vi "TestSortedRecipeFOlderData.vi"() -> ()   [LabVIEW 2022 SP3]
uses:
  Controls/RecipesFolderSummary--Cluster.ctl
  Controls/DLP RecipeTypesData--Cluster.ctl
  Controls/RecipeInfo--Cluster.ctl
panel:
  out "Type":string
  in  "error in (no error)":errorcluster
  in  "OK":bool
  out "found":bool
  in  "RecipeFolderPath":path
  in  "Recipe":u16(ring) items=["25x29 Token Recipe DOE001"]
  in  "Product":u16(ring) items=["25x29 Token", "C30v3.2"]
  in  "RecipeType":u16(ring) items=["PrintDesign", "Calibration"]
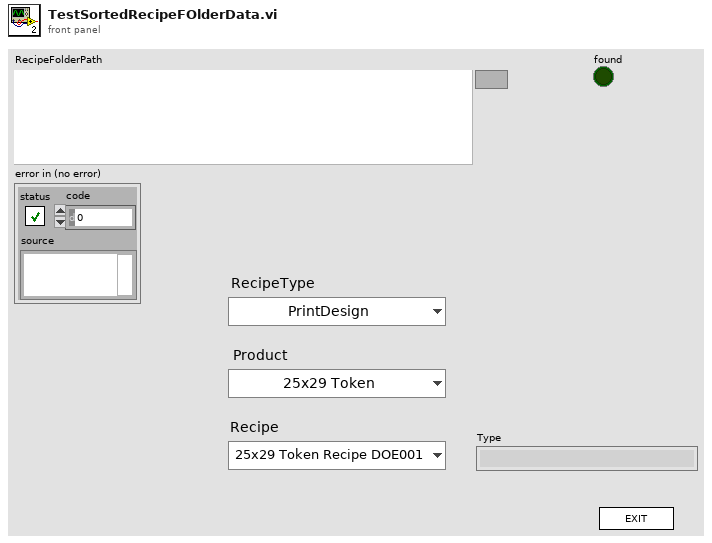
[diagram p1: front panel]
types:
  T1 = typedef "RecipesFolderSummary--Cluster.ctl" = cluster{"Products":string[], "RecipeTypes":string[]}
  T2 = typedef "TD Dynamic CVT DVR--ref.ctl" = refnum<data-value>
  T3 = enum32{"Invalid", "Standard", "Closed", "Hidden", "Minimized", "Maximized"}
  T4 = enum32{"invalid app kind", "Development System", "Run Time System", "Student Edition", "Embedded LabVIEW", "Evaluation", "Custom"}
  T5 = cluster{"Core":cluster{"Current VI Reference":refnum<vi>, "Close Panel on Exit?":bool}, "Your Boolean data":bool, "dCVT DVR out":T2}
  T6 = cluster{"Current VI Reference":refnum<vi>, "Close Panel on Exit?":bool}
  T7 = typedef "DLP RecipeTypesData--Cluster.ctl" = cluster{"Product":string, "RecipePathsByProduct":path[], "RecipeNamesByProduct":string[]}
  T8 = typedef "RecipeInfo--Cluster.ctl" = cluster{"Path":path, "Type":string}
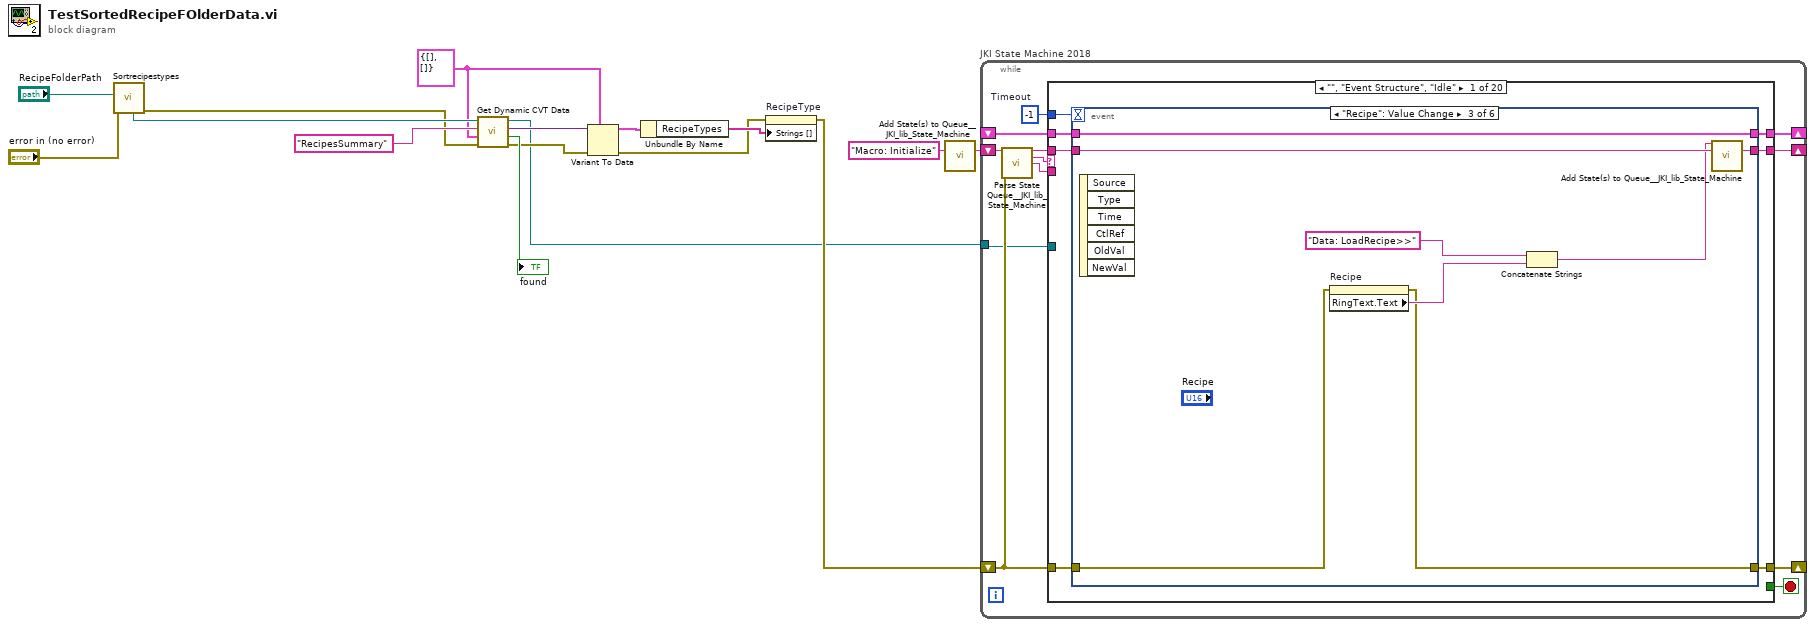
[diagram p0: block diagram]
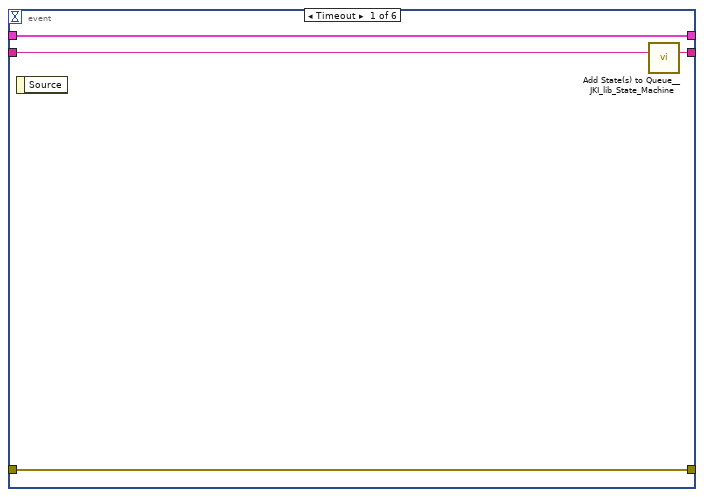
[diagram p2: hidden frame]
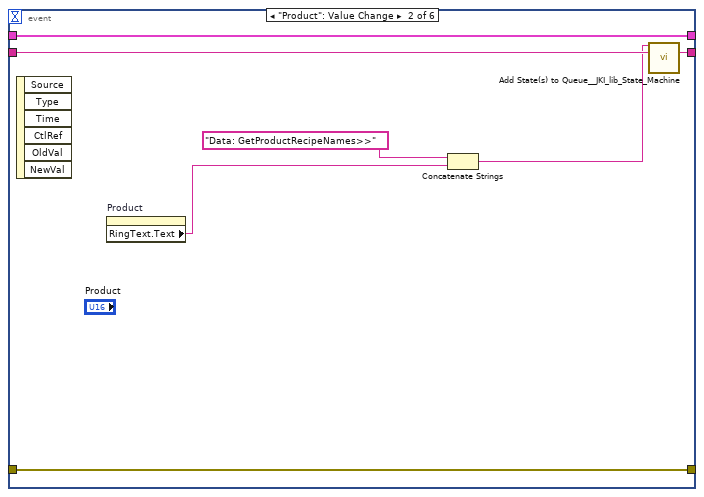
[diagram p3: hidden frame]
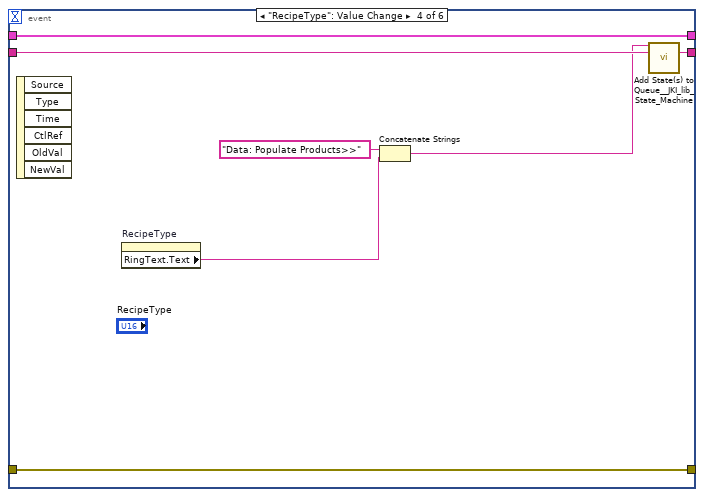
[diagram p4: hidden frame]
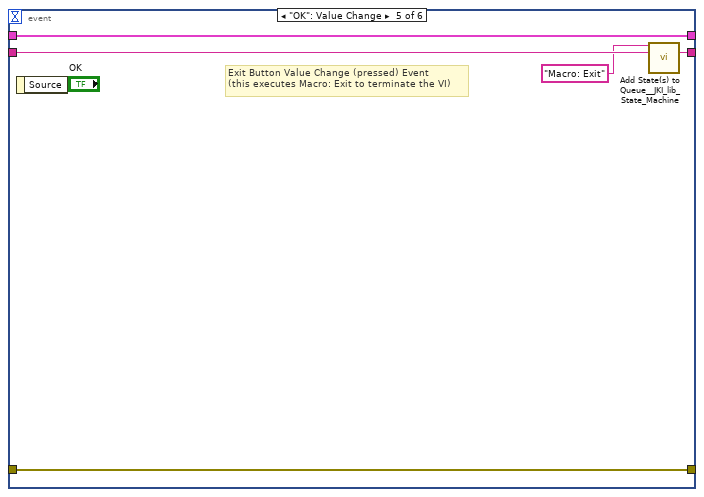
[diagram p5: hidden frame]
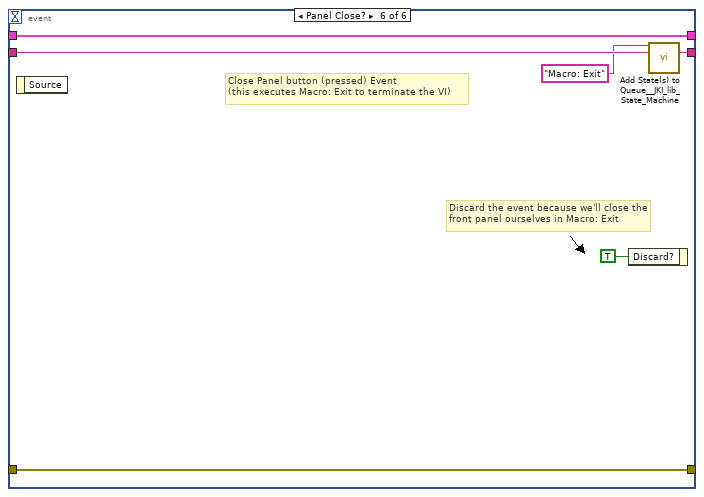
[diagram p6: hidden frame]
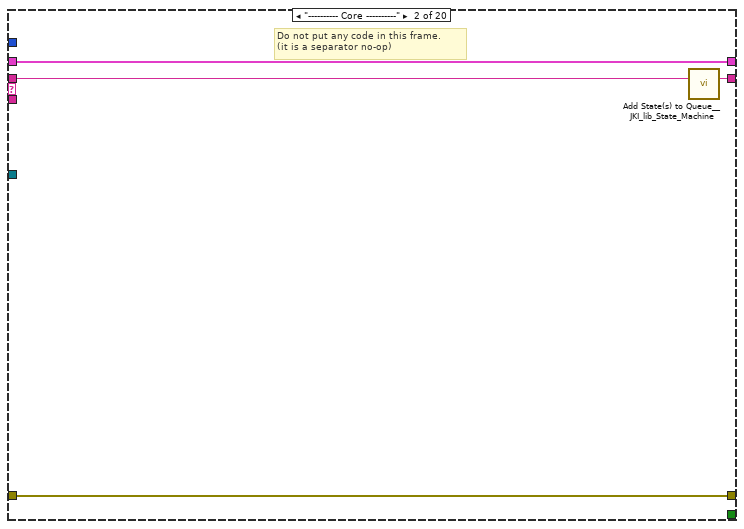
[diagram p7: hidden frame]
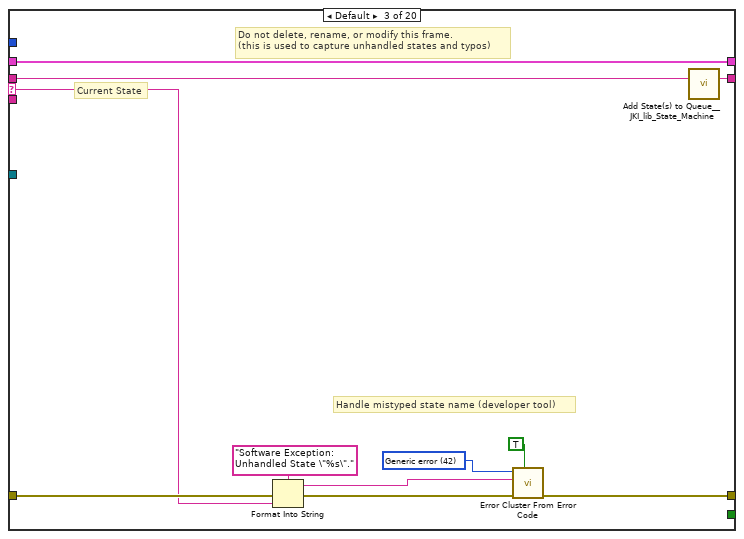
[diagram p8: hidden frame]
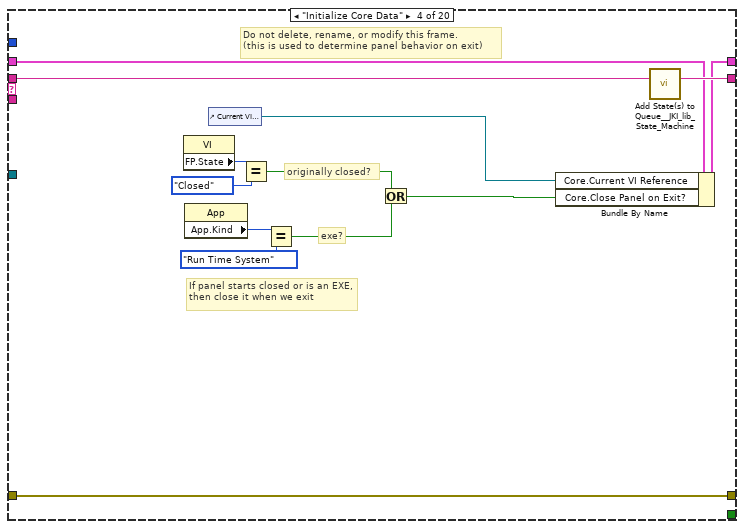
[diagram p9: hidden frame]
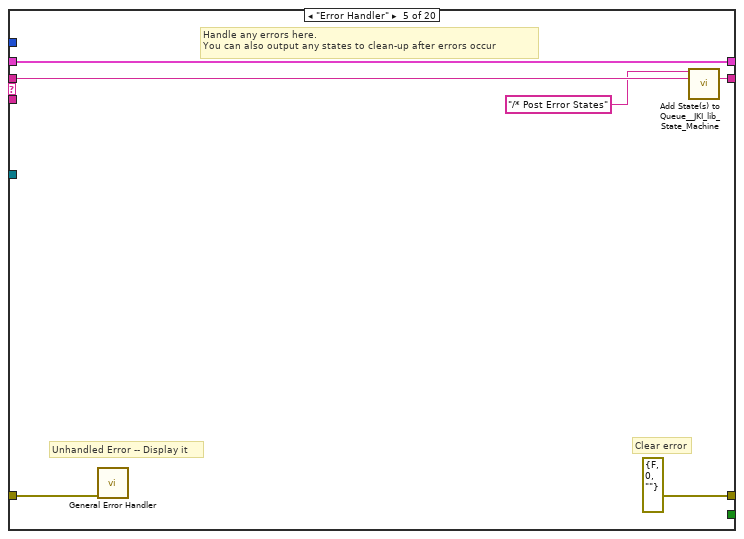
[diagram p10: hidden frame]
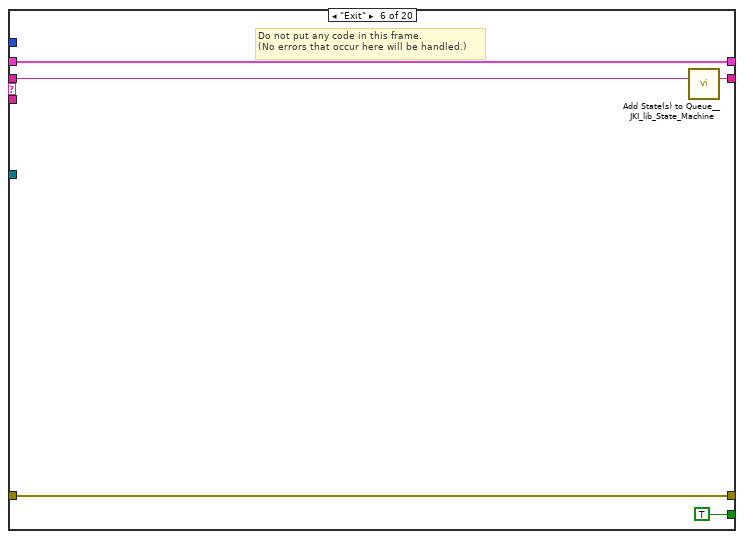
[diagram p11: hidden frame]
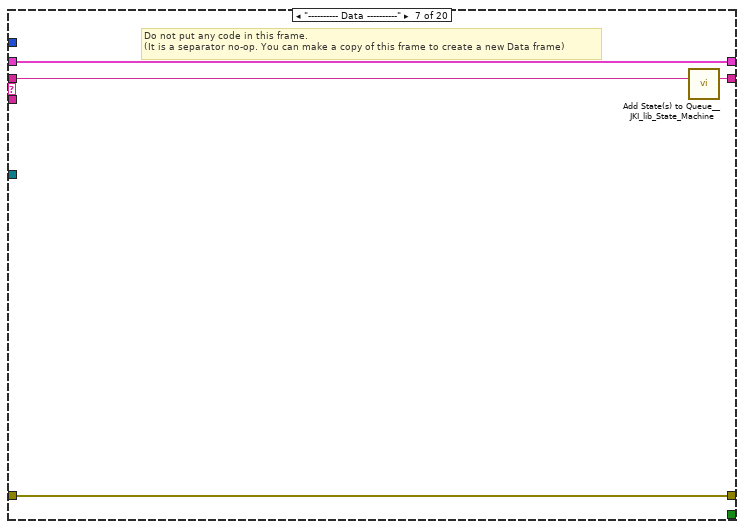
[diagram p12: hidden frame]
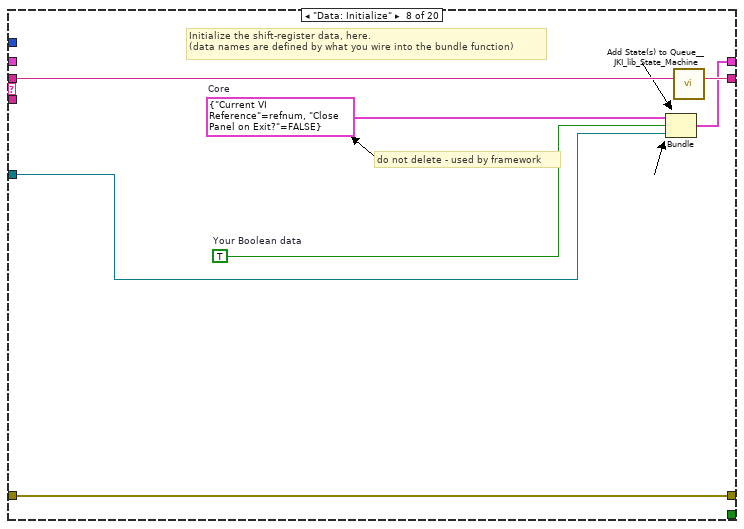
[diagram p13: hidden frame]
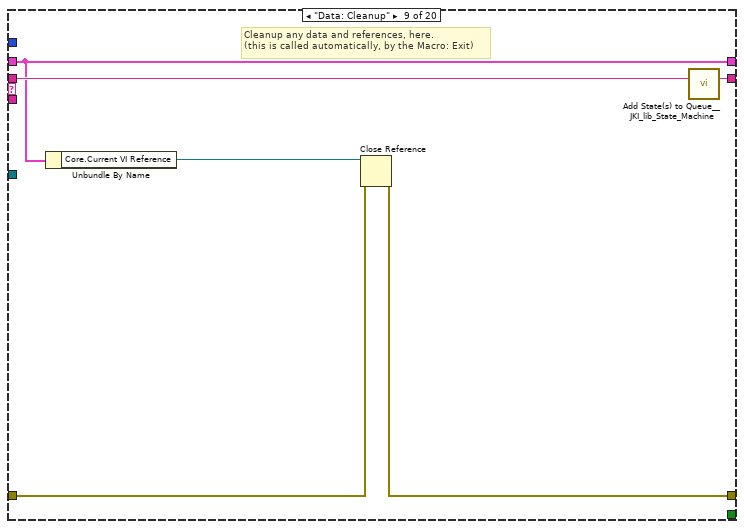
[diagram p14: hidden frame]
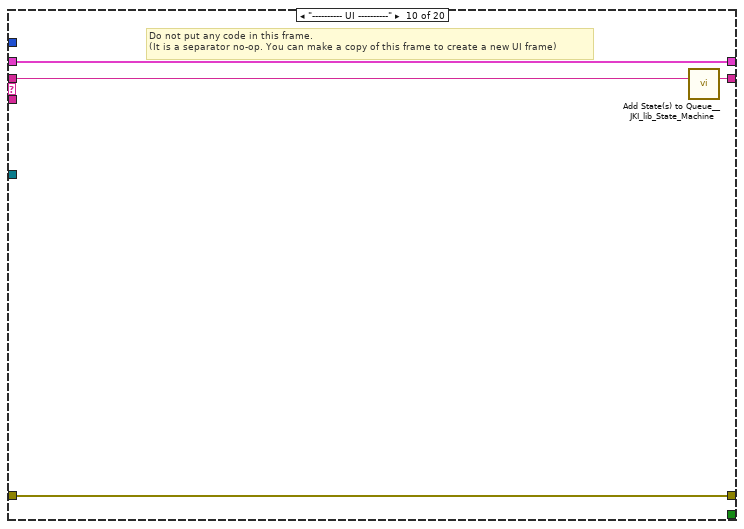
[diagram p15: hidden frame]
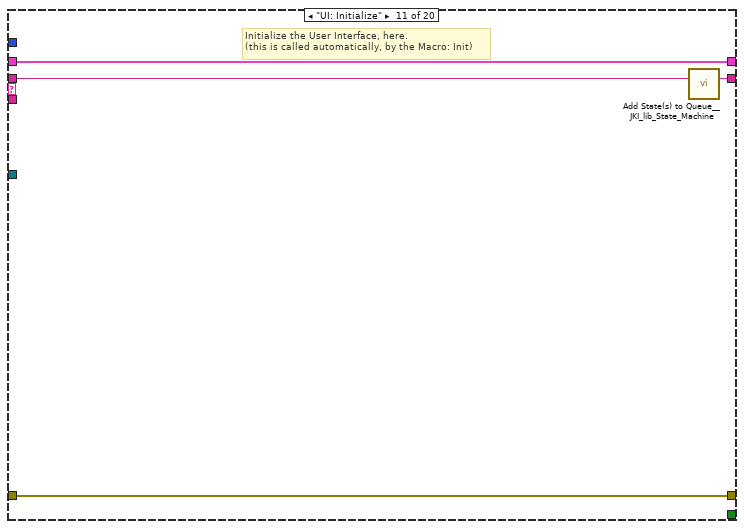
[diagram p16: hidden frame]
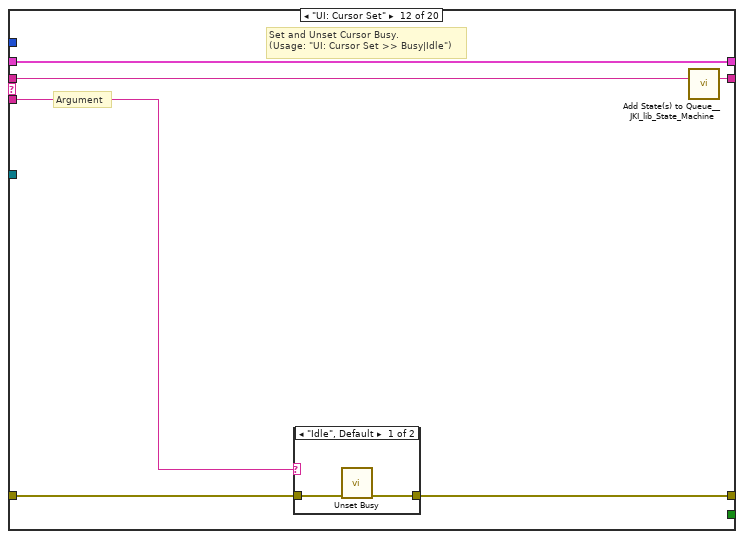
[diagram p17: hidden frame]
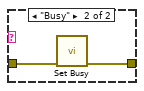
[diagram p18: hidden frame]
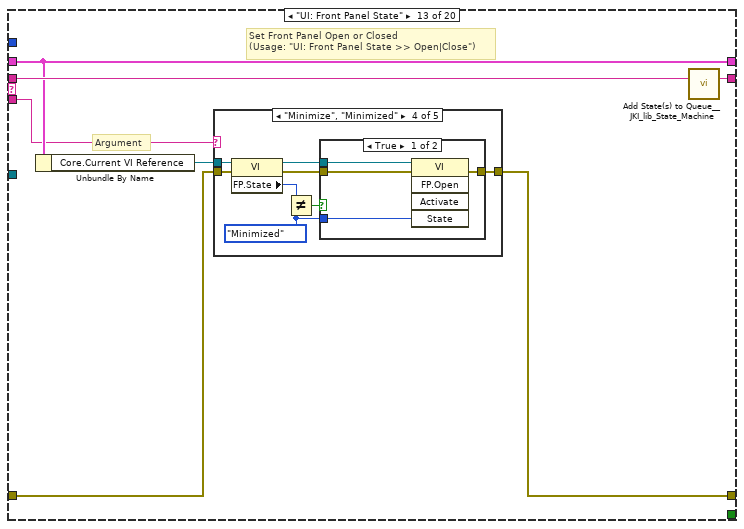
[diagram p19: hidden frame]
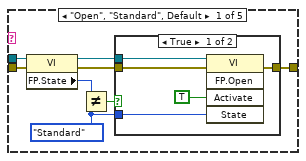
[diagram p20: hidden frame]
diagram:
  w11 = T1 {"Products"=[], "RecipeTypes"=[]}
  n1 = call "Sortrecipestypes.vi"("error in (no error)"="error in (no error)", "RecipeFolderPath"="RecipeFolderPath") -> ("error out"=w2:errorcluster, "DebugDict"=w14:T2)  [unwired: 5 in, 3 out]
  n2 = call <vilib>:"Get Dynamic CVT Data.vi"("error in (no error)"=w2, "default value (empty variant)"=w11, "DataName"="RecipesSummary", "dCVT DVR"=w14) -> ("error out"=w10:errorcluster, "found"=→"found":bool, "value"=w12:variant, "dCVT DVR out"=w4:T2)  [unwired: 4 in]
  n3 = Variant To Data(error in=w10, type=w11, Variant=w12) -> (data=w9:T1, error out=w3:errorcluster)
  n4 = Unbundle By Name(w9) -> ("RecipeTypes"=w8:string[])
  n5 = property on="RecipeType" class="Ring (strict)"(error in=w3, "Strings []"=w8) -> (error out=w5:errorcluster)  [unwired: 1 in, 1 out]
  n6 = call <vilib>:"Add State(s) to Queue__JKI_lib_State_Machine.vi"("State(s) in (\"\")"="Macro: Initialize") -> ("States Out"=w7:string)  [unwired: 14 in]
  n7 = while "JKI State Machine 2018" {
    shift-right: [w21] -> _
    shift-left: _ -> [w20]
    shift-right: [w24] -> _
    shift-left: w5 -> [w18]
    shift-right: [w23] -> _
    shift-left: w7 -> [w25]
    tunnel: w4 -> [w17]
    stop <- w22 stop-if-true
    w19 = -1  # Timeout
    n8 = call <vilib>:"Parse State Queue__JKI_lib_State_Machine.vi"("State Queue"=w25, "Error In (no error)"=w18) -> ("Remaining States"=w27:string, "Current State"=w28:string, "Arguments"=w26:string)  [unwired: 11 in]
    n9 = case shown="\"\", \"Event Structure\", \"Idle\"" w28 {
      selector: w28 -> [_ _ w77 _ _ _ _ _ _ _ _ _ _ _ _ _ _ _ _ _]
      tunnel: w27 -> [w35 w76 w81 w100 w106 w111 w115 w122 w128 w132 w136 w142 w153 w222 w227 w237 w241 w254 w268 w282]
      tunnel: w26 -> [_ _ _ _ _ _ _ _ _ _ _ w137 w147 _ _ _ _ w248 w263 w276]
      tunnel: w20 -> [w33 w73 w79 w93 w103 w109 w112 _ w123 w129 w134 w140 w149 w219 w224 w234 w238 w249 w266 w277]
      tunnel: [w32 w74 w83 w97 errorcluster {"status"=FALSE, "code"=0, "source"=""} ("error out") w108 w113 w119 w124 w130 w133 w138 w150 w220 w225 w235 w239 w243 w255 w269] -> w24
      tunnel: w18 -> [w31 w74 w82 w97 w102 w108 w113 w119 w125 w130 w133 w139 w151 w220 w225 w235 w239 w242 w261 w272]
      tunnel: [w34 w75 w80 w99 w105 w110 w114 w121 w127 w131 w135 w141 w152 w221 w226 w236 w240 w253 w267 w281] -> w23
      tunnel: [_ _ _ _ _ TRUE _ _ _ _ _ _ _ _ _ _ _ _ _ _] -> w22
      tunnel: [w30 w73 w79 w98 w103 w109 w112 w120 w123 w129 w134 w140 w149 w219 w224 w234 w238 w249 w266 w277] -> w21
      tunnel: w19 -> [w29 _ _ _ _ _ _ _ _ _ _ _ _ _ _ _ _ _ _ _]
      tunnel: w17 -> [_ _ _ _ _ _ _ w116 _ _ _ _ _ _ _ _ _ _ _ _]
      frame "", "Event Structure", "Idle" {
        n10 = event shown="[2] \"Recipe\": Value Change" {
          selector: _ -> [_ _ _ _ _ _]
          dyn-events: _ -> [_ _ _ _ _ _]
          timeout: w29 -> [_ _ _ _ _ _]
          tunnel: w35 -> [w39 w46 w54 w61 w66 w72]
          tunnel: [w38 w45 w53 w60 w65 w71] -> w34
          tunnel: w33 -> [w36 w43 w52 w58 w63 w69]
          tunnel: [w37 w44 w48 w59 w64 w70] -> w32
          tunnel: w31 -> [w37 w44 w47 w59 w64 w70]
          tunnel: [w36 w43 w52 w58 w63 w69] -> w30
          event Timeout {
            n11 = event-data() -> ()  [unwired: 1 in, 1 out]
            n12 = call <vilib>:"Add State(s) to Queue__JKI_lib_State_Machine.vi"("State(s) in (\"\")"=w39) -> ("States Out"=w38:string)  [unwired: 14 in]
          }
          event "Product": Value Change {
            n13 = event-data() -> ()  [unwired: 1 in, 6 out]
            n14 = property on="Product" class="Ring (strict)"() -> ("RingText.Text"=w42:string)  [unwired: 2 in, 2 out]
            n15 = Concatenate Strings("Data: GetProductRecipeNames>>" ("string"), w42) -> (w40:string)
            n16 = call <vilib>:"Add State(s) to Queue__JKI_lib_State_Machine.vi"("State(s) in Front (\"\")"=w40, "State(s) in (\"\")"=w46) -> ("States Out"=w45:string)  [unwired: 13 in]
          }
          event "Recipe": Value Change {
            n17 = event-data() -> ()  [unwired: 1 in, 6 out]
            n18 = property on="Recipe" class="Ring (strict)"(error in=w47) -> (error out=w48:errorcluster, "RingText.Text"=w51:string)  [unwired: 1 in, 1 out]
            n19 = Concatenate Strings("Data: LoadRecipe>>" ("string"), w51) -> (w49:string)
            n20 = call <vilib>:"Add State(s) to Queue__JKI_lib_State_Machine.vi"("State(s) in Front (\"\")"=w49, "State(s) in (\"\")"=w54) -> ("States Out"=w53:string)  [unwired: 13 in]
          }
          event "RecipeType": Value Change {
            n21 = event-data() -> ()  [unwired: 1 in, 6 out]
            n22 = property on="RecipeType" class="Ring (strict)"() -> ("RingText.Text"=w56:string)  [unwired: 2 in, 2 out]
            n23 = Concatenate Strings("Data: Populate Products>>" ("string"), w56) -> (w55:string)
            n24 = call <vilib>:"Add State(s) to Queue__JKI_lib_State_Machine.vi"("State(s) in Front (\"\")"=w55, "State(s) in (\"\")"=w61) -> ("States Out"=w60:string)  [unwired: 13 in]
          }
          event "OK": Value Change {
            # "Exit Button Value Change (pressed) Event\n(this executes Macro: Exit to terminate the VI)"
            n25 = event-data() -> ()  [unwired: 1 in, 1 out]
            n26 = call <vilib>:"Add State(s) to Queue__JKI_lib_State_Machine.vi"("State(s) in Front (\"\")"="Macro: Exit", "State(s) in (\"\")"=w66) -> ("States Out"=w65:string)  [unwired: 13 in]
          }
          event Panel Close? {
            # "Discard the event because we'll close the front panel ourselves in Macro: Exit"
            # "Close Panel button (pressed) Event\n(this executes Macro: Exit to terminate the VI)"
            n27 = event-data() -> ()  [unwired: 1 in, 1 out]
            n28 = event-data("Discard?"=TRUE) -> ()  [unwired: 1 in, 1 out]
            n29 = call <vilib>:"Add State(s) to Queue__JKI_lib_State_Machine.vi"("State(s) in Front (\"\")"="Macro: Exit", "State(s) in (\"\")"=w72) -> ("States Out"=w71:string)  [unwired: 13 in]
          }
        }
      }
      frame "---------- Core ----------" {
        # "Do not put any code in this frame.\n(it is a separator no-op)"
        n30 = call <vilib>:"Add State(s) to Queue__JKI_lib_State_Machine.vi"("State(s) in (\"\")"=w76) -> ("States Out"=w75:string)  [unwired: 14 in]
      }
      frame Default {
        w86 = 42 items=["No error", "Argument error", "Memory is full", "Out of zone", "End of file", "File already open", "Generic file I/O error", "File not found", "File permission error", "Disk is full", "Duplicate path", "Too many files open", "System feature not enabled", "Resource file not found", "Cannot add resource", "Resource not found", "Image not found", "Image memory error", "Pen does not exist", "Config type invalid", "Config token not found", "Config parse error", "Config memory error", "Bad external code format", "Bad external code offset", "External code not present", "Null window", "Destroy window error", "Null menu", "Print aborted", "Bad print record", "Print driver error", "Windows error during printing", "Memory error during printing", "Print dialog error", "Generic print error", "Invalid device refnum", "Device not found", "Device parameter error", "Device unit error", "Cannot open device", "Device call aborted", "Generic error", "Cancelled by user", "Object ID too low", "Object ID too high", "Object not in heap", "Unknown heap", "Unknown object (invalid DefProc)", "Unknown object (DefProc not in table)", "Message out of range", "Invalid (null) method", "Unknown message", "Manager call not supported", "Bad address", "Network operation in progress", "Network operation timed out", "Connection is busy", "Network attribute not supported", "Network error", "Address in use", "System out of memory", "Connection aborted", "Connection refused", "Not connected", "Already connected", "Connection closed", "Initialization error (interapplication manager)", "Bad occurrence", "Wait on unbound occurrence handler", "Occurrence queue overflow", "Datalog type conflict", "Unused", "Unrecognized type (interapplication manager)", "Memory corrupt", "Failed to make temporary DLL", "Old CIN version", "Drag socket not found", "Failed to load drop-object", "Failed to register OLE object", "Failed to release OLE object", "Format specifier type mismatch", "Unknown format specifier", "Too few format specifiers", "Too many format specifiers", "Scan failed", "Newer CIN version", "Error converting to variant", "Runtime menu error", "Password tampered", "Variant attribute not found", "Incompatible variant data type", "Event data is not available", "Event Store is not present", "Occurrence is not found", "Event Queue is not created", "Event info is not available", "Refnum passed is NULL", "Error retrieving Class GUID", "Error retrieving CoClass GUID", "Error retrieving TypeLib GUID.", "Bad built application magic bytes.", "Specific driver is different from the specific driver associated with the Logical Name.", "There is no session opened to the class driver.", "Max Error", "MAX - Error with config objects", "MAX - Error loading configuration", "MAX - Group not supported"]
        # "Current State"
        # "Do not delete, rename, or modify this frame.\n(this is used to capture unhandled states and typos)"
        # "Handle mistyped state name (developer tool)"
        n31 = Format Into String(format string="Software Exception: Unhandled State \"%s\"." ("message"), error in=w82, w77) -> (resulting string=w85:string, error out=w84:errorcluster)  [unwired: 1 in]
        n32 = call <vilib>:"Error Cluster From Error Code.vi"("show call chain? (False)"=TRUE, "error in (no error)"=w84, "error message (\"\")"=w85, "error code (0)"=w86) -> ("error out"=w83:errorcluster)  [unwired: 5 in]
        n33 = call <vilib>:"Add State(s) to Queue__JKI_lib_State_Machine.vi"("State(s) in (\"\")"=w81) -> ("States Out"=w80:string)  [unwired: 14 in]
      }
      frame "Initialize Core Data" {
        # "Do not delete, rename, or modify this frame.\n(this is used to determine panel behavior on exit)"
        # "originally closed?"
        # "exe?"
        # "If panel starts closed or is an EXE, then close it when we exit"
        n34 = property class="VI"() -> ("FP.State"=w90:T3)  [unwired: 2 in, 2 out]
        n35 = property class="App"() -> ("App.Kind"=w96:T4)  [unwired: 2 in, 2 out]
        n36 = control-ref of="Current VI Reference"() -> (w91:refnum<vi>)
        n37 = Equal?(x=w90, y=T3."Closed" ("Front Panel Window:State")) -> (x = y?=w88:bool)
        n38 = Equal?(x=w96, y=T4."Run Time System" ("Application:Kind")) -> (x = y?=w94:bool)
        n39 = Or(x=w88, y=w94) -> (x .or. y?=w92:bool)
        n40 = Bundle By Name(cluster=w93, "Core.Current VI Reference"=w91, "Core.Close Panel on Exit?"=w92) -> (w98:T5)
        n41 = call <vilib>:"Add State(s) to Queue__JKI_lib_State_Machine.vi"("State(s) in (\"\")"=w100) -> ("States Out"=w99:string)  [unwired: 14 in]
      }
      frame "Error Handler" {
        # "Unhandled Error -- Display it"
        # "Handle any errors here.\nYou can also output any states to clean-up after errors occur"
        # "Clear error"
        n42 = call <vilib>:"General Error Handler.vi"("error in (no error)"=w102) -> ()  [unwired: 10 in, 5 out]
        n43 = call <vilib>:"Add State(s) to Queue__JKI_lib_State_Machine.vi"("State(s) in Front (\"\")"="/* Post Error States", "State(s) in (\"\")"=w106) -> ("States Out"=w105:string)  [unwired: 13 in]
      }
      frame "Exit" {
        # "Do not put any code in this frame.\n(No errors that occur here will be handled.)"
        n44 = call <vilib>:"Add State(s) to Queue__JKI_lib_State_Machine.vi"("State(s) in (\"\")"=w111) -> ("States Out"=w110:string)  [unwired: 14 in]
      }
      frame "---------- Data ----------" {
        # "Do not put any code in this frame.\n(It is a separator no-op. You can make a copy of this frame to create a new Data frame)"
        n45 = call <vilib>:"Add State(s) to Queue__JKI_lib_State_Machine.vi"("State(s) in (\"\")"=w115) -> ("States Out"=w114:string)  [unwired: 14 in]
      }
      frame "Data: Initialize" {
        w117 = T6 {"Current VI Reference"=refnum, "Close Panel on Exit?"=FALSE}  # Core
        w118 = TRUE  # Your Boolean data
        # "do not delete - used by framework"
        # "Initialize the shift-register data, here.\n(data names are defined by what you wire into the bundle function)"
        n46 = Bundle("Core"=w117, "Your Boolean data"=w118, "dCVT DVR out"=w116) -> (w120:T5)  [unwired: 1 in]
        n47 = call <vilib>:"Add State(s) to Queue__JKI_lib_State_Machine.vi"("State(s) in (\"\")"=w122) -> ("States Out"=w121:string)  [unwired: 14 in]
      }
      frame "Data: Cleanup" {
        # "Cleanup any data and references, here.\n(this is called automatically, by the Macro: Exit)"
        n48 = Unbundle By Name(w123) -> ("Core.Current VI Reference"=w126:refnum<vi>)
        n49 = Close Reference(reference=w126, error in (no error)=w125) -> (error out=w124:errorcluster)
        n50 = call <vilib>:"Add State(s) to Queue__JKI_lib_State_Machine.vi"("State(s) in (\"\")"=w128) -> ("States Out"=w127:string)  [unwired: 14 in]
      }
      frame "---------- UI ----------" {
        # "Do not put any code in this frame.\n(It is a separator no-op. You can make a copy of this frame to create a new UI frame)"
        n51 = call <vilib>:"Add State(s) to Queue__JKI_lib_State_Machine.vi"("State(s) in (\"\")"=w132) -> ("States Out"=w131:string)  [unwired: 14 in]
      }
      frame "UI: Initialize" {
        # "Initialize the User Interface, here.\n(this is called automatically, by the Macro: Init)"
        n52 = call <vilib>:"Add State(s) to Queue__JKI_lib_State_Machine.vi"("State(s) in (\"\")"=w136) -> ("States Out"=w135:string)  [unwired: 14 in]
      }
      frame "UI: Cursor Set" {
        # "Argument"
        # "Set and Unset Cursor Busy.\n(Usage: \"UI: Cursor Set >> Busy|Idle\")"
        n53 = case shown="\"Idle\", Default" w137 {
          tunnel: w139 -> [w144 w146]
          tunnel: [w143 w145] -> w138
          frame "Idle", Default {
            n54 = call <vilib>:"Unset Busy.vi"("error in (no error)"=w144) -> ("error out"=w143:errorcluster)  [unwired: 10 in]
          }
          frame "Busy" {
            n55 = call <vilib>:"Set Busy.vi"("error in (no error)"=w146) -> ("error out"=w145:errorcluster)  [unwired: 9 in, 1 out]
          }
        }
        n56 = call <vilib>:"Add State(s) to Queue__JKI_lib_State_Machine.vi"("State(s) in (\"\")"=w142) -> ("States Out"=w141:string)  [unwired: 14 in]
      }
      frame "UI: Front Panel State" {
        # "Argument"
        # "Set Front Panel Open or Closed\n(Usage: \"UI: Front Panel State >> Open|Close\")"
        n57 = Unbundle By Name(w149) -> ("Core.Current VI Reference"=w148:refnum<vi>)
        n58 = case shown="\"Minimize\", \"Minimized\"" w147 {
          tunnel: w151 -> [w159 w174 w185 w198 w211]
          tunnel: [w161 w175 w187 w200 w213] -> w150
          tunnel: w148 -> [w160 w172 w186 w199 w212]
          frame "Open", "Standard", Default {
            w154 = T3."Standard" ("State")
            n59 = property class="VI"(reference=w160, error in=w159) -> (reference out=w157:refnum<vi>, error out=w158:errorcluster, "FP.State"=w156:T3)
            n60 = Not Equal?(x=w156, y=w154) -> (x != y?=w155:bool)
            n61 = case shown="True" w155 {
              tunnel: [w165 w167] -> w161
              tunnel: w158 -> [w164 w167]
              tunnel: w157 -> [w163 _]
              tunnel: w154 -> [w162 _]
              frame True {
                n62 = invoke class="VI" method="FP.Open"(reference=w163, error in=w164, "Activate"=TRUE, "State"=w162) -> (error out=w165:errorcluster)  [unwired: 1 in, 4 out]
              }
              frame False {
              }
            }
          }
          frame "Close", "Closed" {
            n63 = property class="VI"(reference=w172, error in=w174) -> (reference out=w171:refnum<vi>, error out=w173:errorcluster, "FP.State"=w169:T3)
            n64 = Not Equal?(x=w169, y=T3."Closed" ("Front Panel Window:State")) -> (x != y?=w168:bool)
            n65 = case shown="True" w168 {
              tunnel: [w176 w179] -> w175
              tunnel: w173 -> [w176 w178]
              tunnel: w171 -> [_ w177]
              frame False {
              }
              frame True {
                n66 = invoke class="VI" method="FP.Close"(reference=w177, error in=w178) -> (error out=w179:errorcluster)  [unwired: 1 in, 2 out]
              }
            }
          }
          frame "Hidden", "Hide" {
            w180 = T3."Hidden" ("State")
            n67 = property class="VI"(reference=w186, error in=w185) -> (reference out=w183:refnum<vi>, error out=w184:errorcluster, "FP.State"=w182:T3)
            n68 = Not Equal?(x=w182, y=w180) -> (x != y?=w181:bool)
            n69 = case shown="True" w181 {
              tunnel: [w191 w192] -> w187
              tunnel: w184 -> [w190 w192]
              tunnel: w183 -> [w189 _]
              tunnel: w180 -> [w188 _]
              frame True {
                n70 = invoke class="VI" method="FP.Open"(reference=w189, error in=w190, "State"=w188) -> (error out=w191:errorcluster)  [unwired: 2 in, 4 out]
              }
              frame False {
              }
            }
          }
          frame "Minimize", "Minimized" {
            w193 = T3."Minimized" ("State")
            n71 = property class="VI"(reference=w199, error in=w198) -> (reference out=w196:refnum<vi>, error out=w197:errorcluster, "FP.State"=w195:T3)
            n72 = Not Equal?(x=w195, y=w193) -> (x != y?=w194:bool)
            n73 = case shown="True" w194 {
              tunnel: [w204 w205] -> w200
              tunnel: w197 -> [w203 w205]
              tunnel: w196 -> [w202 _]
              tunnel: w193 -> [w201 _]
              frame True {
                n74 = invoke class="VI" method="FP.Open"(reference=w202, error in=w203, "State"=w201) -> (error out=w204:errorcluster)  [unwired: 2 in, 4 out]
              }
              frame False {
              }
            }
          }
          frame "Maximize", "Maximized" {
            w206 = T3."Maximized" ("State")
            n75 = property class="VI"(reference=w212, error in=w211) -> (reference out=w209:refnum<vi>, error out=w210:errorcluster, "FP.State"=w208:T3)
            n76 = Not Equal?(x=w208, y=w206) -> (x != y?=w207:bool)
            n77 = case shown="True" w207 {
              tunnel: [w217 w218] -> w213
              tunnel: w210 -> [w216 w218]
              tunnel: w209 -> [w215 _]
              tunnel: w206 -> [w214 _]
              frame True {
                n78 = invoke class="VI" method="FP.Open"(reference=w215, error in=w216, "State"=w214) -> (error out=w217:errorcluster)  [unwired: 2 in, 4 out]
              }
              frame False {
              }
            }
          }
        }
        n79 = call <vilib>:"Add State(s) to Queue__JKI_lib_State_Machine.vi"("State(s) in (\"\")"=w153) -> ("States Out"=w152:string)  [unwired: 14 in]
      }
      frame "---------- Macro ----------" {
        # "Do not put any code in this frame.\n(It is a separator no-op. You can make a copy of this frame to create a new Macro frame)"
        n80 = call <vilib>:"Add State(s) to Queue__JKI_lib_State_Machine.vi"("State(s) in (\"\")"=w222) -> ("States Out"=w221:string)  [unwired: 14 in]
      }
      frame "Macro: Initialize" {
        w223 = "Data: Initialize\nInitialize Core Data\nUI: Initialize\nUI: Front Panel State >> Open"  # Data: Initialize Initialize Core Data UI: Initialize UI: Front Panel State >> Open
        # "Initialization Macro\n(This is called once, when the VI starts)"
        n81 = call <vilib>:"Add State(s) to Queue__JKI_lib_State_Machine.vi"("State(s) in Front (\"\")"=w223, "State(s) in (\"\")"=w227) -> ("States Out"=w226:string)  [unwired: 13 in]
      }
      frame "Macro: Exit" {
        # "Exit Macro\n(This is called once, when the VI exits)"
        n82 = Unbundle By Name(w234) -> ("Core.Close Panel on Exit?"=w233:bool)
        n83 = Select(t="UI: Front Panel State >> Close", s=w233, f="") -> (s? t:f=w230:string)
        n84 = call <vilib>:"Add State(s) to Queue__JKI_lib_State_Machine.vi"("State(s) in (\"\")"=w230, "State(s) at Back (\"\")"="Data: Cleanup\nExit") -> ("States Out"=w228:string)  [unwired: 13 in]
        n85 = call <vilib>:"Add State(s) to Queue__JKI_lib_State_Machine.vi"("State(s) in Front (\"\")"=w228, "State(s) in (\"\")"=w237) -> ("States Out"=w236:string)  [unwired: 13 in]
      }
      frame "---------- New Category ----------" {
        # "Template Separator\n(You can make a copy of, or modify, this frame)"
        n86 = call <vilib>:"Add State(s) to Queue__JKI_lib_State_Machine.vi"("State(s) in (\"\")"=w241) -> ("States Out"=w240:string)  [unwired: 14 in]
      }
      frame "Data: GetProductRecipeNames" {
        w247 = T7 {"Product"="", "RecipePathsByProduct"=[], "RecipeNamesByProduct"=[]}
        n87 = Unbundle By Name(w249) -> ("dCVT DVR out"=w252:T2)
        n88 = call <vilib>:"Get Dynamic CVT Data.vi"("error in (no error)"=w242, "default value (empty variant)"=w247, "DataName"=w248, "dCVT DVR"=w252) -> ("error out"=w251:errorcluster, "value"=w250:variant)  [unwired: 4 in, 2 out]
        n89 = Variant To Data(error in=w251, type=w247, Variant=w250) -> (data=w246:T7, error out=w244:errorcluster)
        n90 = Unbundle By Name(w246) -> ("RecipeNamesByProduct"=w245:string[])
        n91 = property on="Recipe" class="Ring (strict)"(error in=w244, "Strings []"=w245) -> (error out=w243:errorcluster)  [unwired: 1 in, 1 out]
        n92 = call <vilib>:"Add State(s) to Queue__JKI_lib_State_Machine.vi"("State(s) in (\"\")"=w254) -> ("States Out"=w253:string)  [unwired: 14 in]
      }
      frame "Data: Populate Products" {
        w258 = string[] [] ("elements")
        n93 = Unbundle By Name(w266) -> ("dCVT DVR out"=w265:T2)
        n94 = Concatenate Strings(w263, "Products" ("string")) -> (w262:string)
        n95 = call <vilib>:"Get Dynamic CVT Data.vi"("error in (no error)"=w261, "default value (empty variant)"=w258, "DataName"=w262, "dCVT DVR"=w265) -> ("error out"=w260:errorcluster, "value"=w259:variant)  [unwired: 4 in, 2 out]
        n96 = Variant To Data(error in=w260, type=w258, Variant=w259) -> (data=w257:string[], error out=w256:errorcluster)
        n97 = property on="Product" class="Ring (strict)"(error in=w256, "Strings []"=w257) -> (error out=w255:errorcluster)  [unwired: 1 in, 1 out]
        n98 = call <vilib>:"Add State(s) to Queue__JKI_lib_State_Machine.vi"("State(s) in (\"\")"=w268) -> ("States Out"=w267:string)  [unwired: 14 in]
      }
      frame "Data: LoadRecipe" {
        w275 = T8 {"Path"=path "", "Type"=""} ("RecipeInfo")
        n99 = Unbundle By Name(w277) -> ("dCVT DVR out"=w280:T2)
        n100 = call <vilib>:"Get Dynamic CVT Data.vi"("error in (no error)"=w272, "default value (empty variant)"=w275, "DataName"=w276, "dCVT DVR"=w280) -> ("error out"=w279:errorcluster, "value"=w278:variant)  [unwired: 4 in, 2 out]
        n101 = Variant To Data(error in=w279, type=w275, Variant=w278) -> (data=w274:T8, error out=w270:errorcluster)
        n102 = Unbundle By Name(w274) -> ("Path"=w271:path, "Type"=w273:string)
        "Type" <- w273
        n103 = case shown="\"PrintDesign\"" w273 {
          tunnel: w271 -> [_ w286 w289]
          tunnel: w270 -> [w283 w285 w288]
          tunnel: [w283 w284 w287] -> w269
          frame Default {
          }
          frame "PrintDesign" {
            n104 = call "DLP_RecipePrints_XML_Read.vi"("error in (no error)"=w285, "Recipe XML File Path"=w286) -> ("error out"=w284:errorcluster)  [unwired: 8 in, 1 out]
          }
          frame "Calibration" {
            n105 = call "DLP_CalibrationPrints_XML_Read.vi"("error in (no error)"=w288, "Recipe XML File Path"=w289) -> ("error out"=w287:errorcluster)  [unwired: 8 in, 1 out]
          }
        }
        n106 = call <vilib>:"Add State(s) to Queue__JKI_lib_State_Machine.vi"("State(s) in (\"\")"=w282) -> ("States Out"=w281:string)  [unwired: 14 in]
      }
    }
  }
